vi "Read Tokens.vi"(8 "error in (no error)":errorcluster, 11 "input string":string) -> (0 "error out":errorcluster, 2 "Token Secret":string, 3 "Token":string)   [LabVIEW 2011, in "i3-oauth.lvlib"]
uses:
  i3-oauth.lvlib
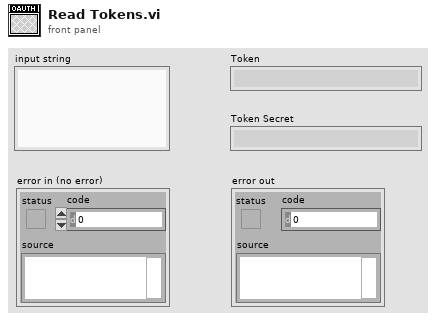
[diagram p1: front panel]
types:
  T1 = typedef "i3-oauth.lvlib/Name-Value Pair.ctl" = cluster{"Name":string, "Value":string}
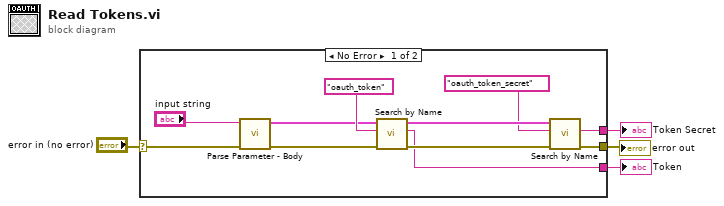
[diagram p0: block diagram]
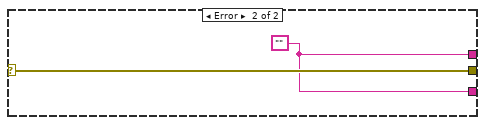
[diagram p2: hidden frame]
diagram:
  n1 = case shown="No Error" "error in (no error)" {
    selector: "error in (no error)" -> [w14 w17]
    tunnel: [w11 w17] -> w4
    tunnel: [w7 w16] -> w2
    tunnel: [w5 w16] -> w1
    frame No Error {
      n2 = call "Parse Parameter - Body.vi"("error in (no error)"=w14, "Body"="input string") -> ("error out"=w13:errorcluster, "Body Parameters"=w9:T1[])  [unwired: 8 in]
      n3 = call "Search by Name.vi"("error in (no error)"=w13, "Name"="oauth_token" ("Key"), "Name-Value Pair List"=w9) -> ("error out"=w12:errorcluster, "Value"=w7:string, "Name-Value Pair List Passthrough"=w8:T1[])  [unwired: 6 in]
      n4 = call "Search by Name.vi"("error in (no error)"=w12, "Name"="oauth_token_secret" ("Key"), "Name-Value Pair List"=w8) -> ("error out"=w11:errorcluster, "Value"=w5:string)  [unwired: 6 in, 1 out]
    }
    frame Error {
      w16 = ""
    }
  }
  "error out" <- w4
  "Token" <- w2
  "Token Secret" <- w1
